vi "Teleop.vi"(10 "Match Info":T1={"Autonomous Elapsed Seconds"=0.0, "TeleOp Elapsed Seconds"=0.0, "Disabled Elapsed Seconds"=0.0, "Visited Autonomous"=FALSE, "Visited TeleOp"=FALSE, "Visited Disabled"=FALSE, "Autonomous Settings"={"Autonomous Style"=enum."Independent", "VI Refnum"=refnum}}, 11 "Call Context":T2) -> ()   [LabVIEW 2011]
doc: "This VI is called for each TeleOp packet received from the DS where the robot is not disabled. It is often used to read from the joysticks and update I/O or to update setpoints for timed control loops. It should complete and return within 20 milliseconds or it may miss DS packets."
uses:
  <vilib>/Rock Robotics/WPI/DriverStation/WPI_DriverStationDerivedRobotMode.ctl
  <vilib>/Rock Robotics/WPI/DriverStation/WPI_DriverStationMatch Info.ctl
  Robot Global Data.vi
panel:
  out "Position 4":dbl
  out "Position 3":dbl
  out "Shift Control":dbl=2.0 format="%.2f"
  in  "Left High":dbl=0.2
  in  "Right High":dbl=0.8
  in  "Left Mid":dbl=0.25
  in  "Right Mid":dbl=0.7
  in  "Shift Input 2":dbl
  in  "Left Low":dbl=0.8
  in  "Right Low":dbl=0.4
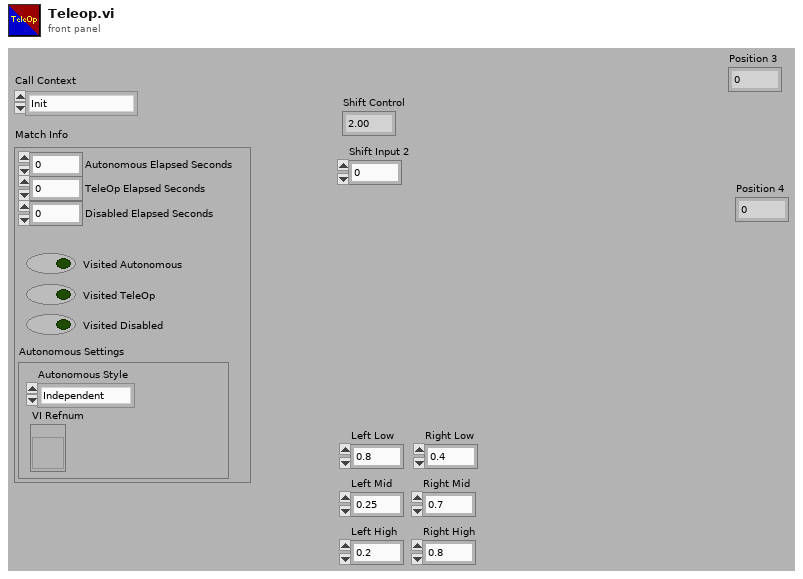
[diagram p1: front panel]
types:
  T1 = typedef "WPI_DriverStationMatch Info.ctl" = cluster{"Autonomous Elapsed Seconds":dbl, "TeleOp Elapsed Seconds":dbl, "Disabled Elapsed Seconds":dbl, "Visited Autonomous":bool, "Visited TeleOp":bool, "Visited Disabled":bool, "Autonomous Settings":cluster{"Autonomous Style":enum16{"Iterative", "Independent"}, "VI Refnum":refnum<vi>}}
  T2 = typedef "WPI_DriverStationDerivedRobotMode.ctl" = enum16{"Init", "Execute", "Stop"}
  T3 = typedef "WPI_MotorControlDeviceRef.ctl" = cluster{"DeviceStatus":errorcluster, "Type":enum16{"PWM", "CAN"}, "PWM":cluster{"Digital Module":T4, "PWM Channel":T5, "DeadBand":T6}, "CAN":cluster{"Device Number":u8, "Control Mode":T7, "Semaphore":T8, "Max Vout":dbl}, "Invert":bool, "TransformRef":T9, "InvTransformRef":T9}
  T4 = typedef "FPGA_TypedefDigitalModule.ctl" = enum16{"Digital Module 1", "Digital Module 2"}
  T5 = typedef "FPGA_DIOPWMChannel.ctl" = enum8{"PWM 1", "PWM 2", "PWM 3", "PWM 4", "PWM 5", "PWM 6", "PWM 7", "PWM 8", "PWM 9", "PWM 10", "Invalid"}
  T6 = typedef "WPI_PWMDeadband.ctl" = cluster{"Name":string, "maxPositivePwm":i32, "minPositivePwm":i32, "centerPwm":i32, "maxNegativePwm":i32, "minNegativePwm":i32, "angularRange":u16}
  T7 = typedef "WPI_CANJaguar_ControlMode.ctl" = enum8{"Percent VBus", "Current", "Speed", "Position", "Voltage"}
  T8 = typedef "Semaphore RefNum" = refnum<k1>
  T9 = typedef "WPI_PWMTransform_ConPane.ctl" = refnum<vi>
  T10 = typedef "WPI_JoystickDevRef.ctl" = cluster{"Device":T11}
  T11 = typedef "WPI_JoystickDeviceEnum.ctl" = enum16{"USB 1", "USB 2", "USB 3", "USB 4", "Kinect 1", "Kinect 2"}
  T12 = typedef "WPI_JoystickButtonState.ctl" = cluster{"Button 1":bool, "Button 2":bool, "Button 3":bool, "Button 4":bool, "Button 5":bool, "Button 6":bool, "Button 7":bool, "Button 8":bool, "Button 9":bool, "Button 10":bool, "Button 11":bool, "Button 12":bool}
  T13 = cluster{"axis 1 (x)":dbl, "axis 2 (y)":dbl, "axis 3 (throttle)":dbl, "axis 4":dbl, "axis 5":dbl, "axis 6":dbl}
  T14 = typedef "WPI_DigitalInputDevRef.ctl" = cluster{"DevStatus":errorcluster, "DIO Channel":T15, "Digital Module":T4}
  T15 = typedef "FPGA_DIOChannel.ctl" = enum8{"DIO 1", "DIO 2", "DIO 3", "DIO 4", "DIO 5", "DIO 6", "DIO 7", "DIO 8", "DIO 9", "DIO 10", "DIO 11", "DIO 12", "DIO 13", "DIO 14", "Invalid"}
  T16 = typedef "WPI_ServoDeviceRef.ctl" = cluster{"DeviceStatus":errorcluster, "Digital Module":T4, "PWM Channel":T5, "DeadBand":T6}
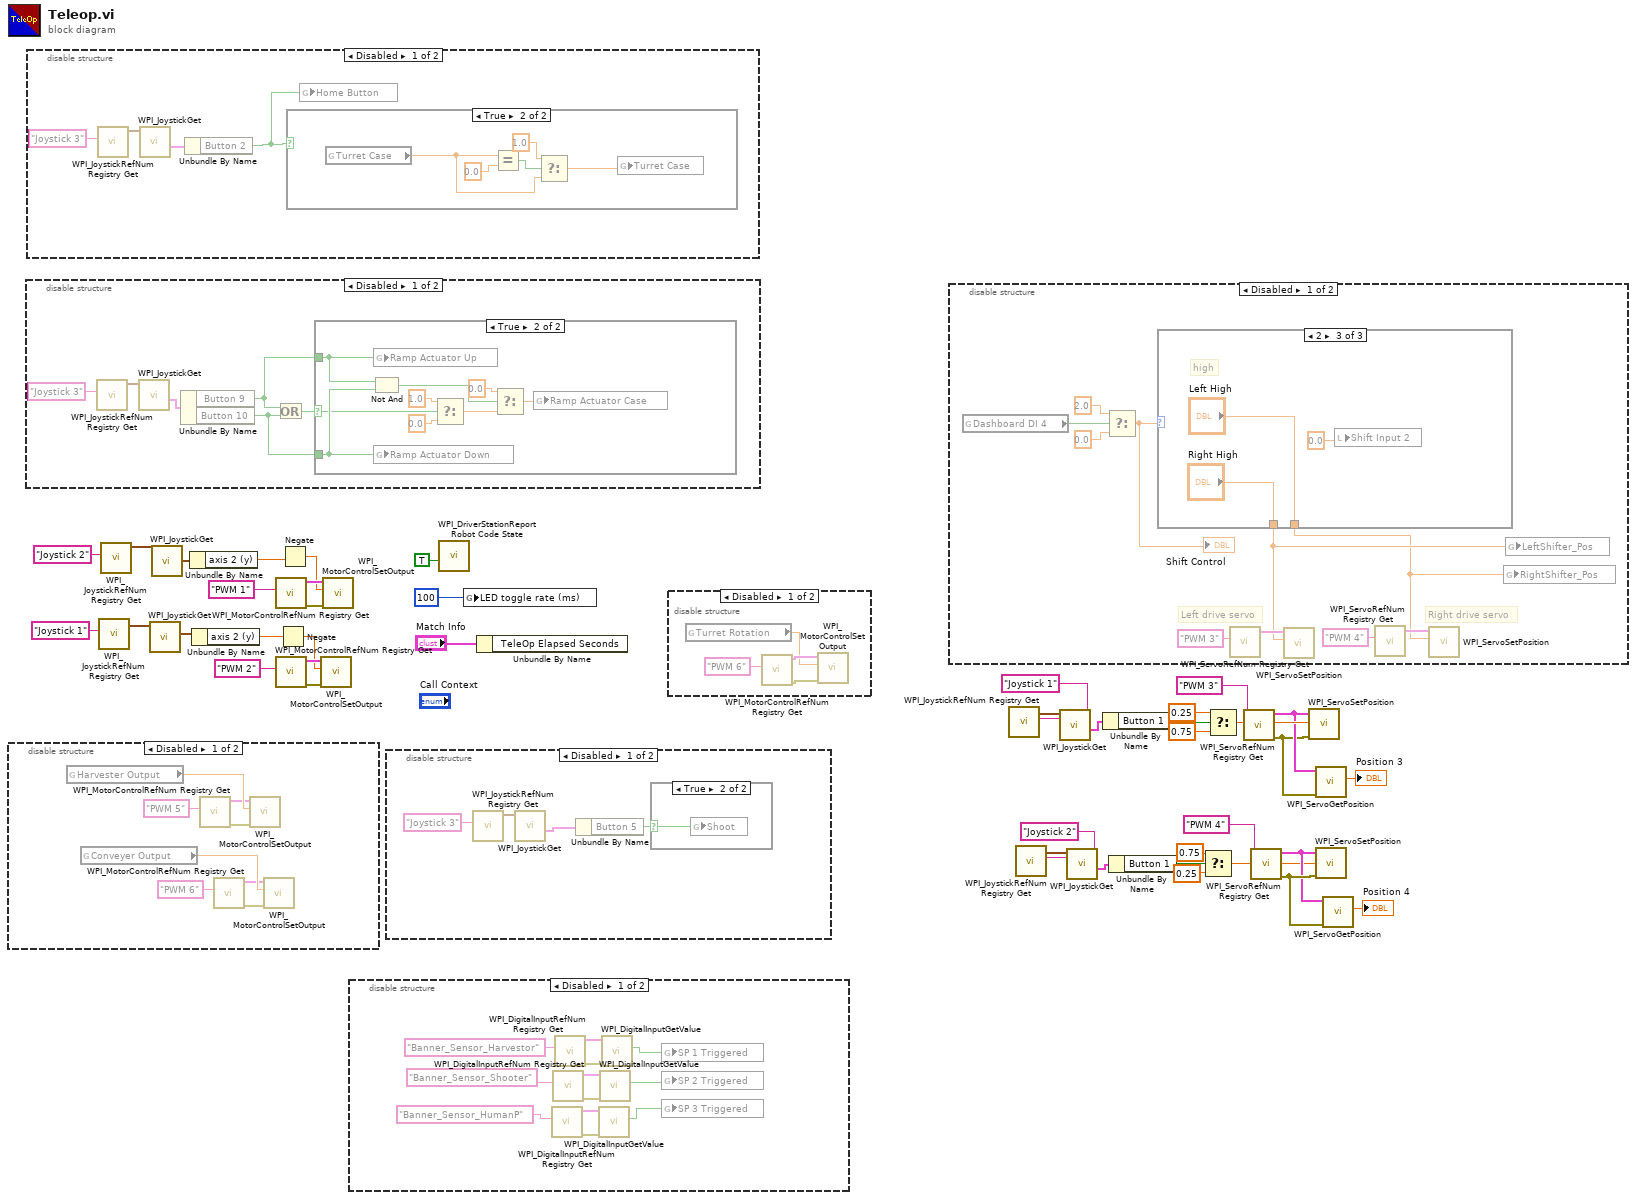
[diagram p0: block diagram]
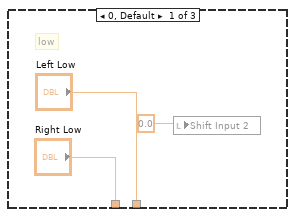
[diagram p11: hidden frame]
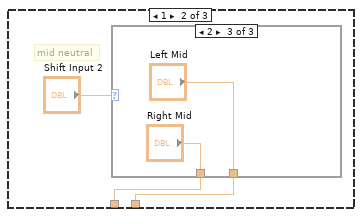
[diagram p12: hidden frame]
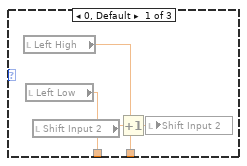
[diagram p13: hidden frame]
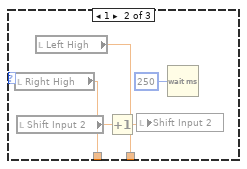
[diagram p14: hidden frame]
diagram:
  n1 = disable-structure shown="Disabled" {
    frame Disabled {
      n2 = global read "Robot Global Data.vi" "Harvester Output"() -> (w47:dbl)
      n3 = global read "Robot Global Data.vi" "Conveyer Output"() -> (w43:dbl)
      n4 = call <vilib>:"WPI_MotorControlRefNum Registry Get.vi"("refnum name"="PWM 5") -> ("error out"=w48:errorcluster, "MotorControlDevRef"=w46:T3)  [unwired: 9 in]
      n5 = call <vilib>:"WPI_MotorControlRefNum Registry Get.vi"("refnum name"="PWM 6") -> ("error out"=w44:errorcluster, "MotorControlDevRef"=w42:T3)  [unwired: 9 in]
      n6 = call <vilib>:"WPI_MotorControlSetOutput.vi"("error in (no error)"=w48, "Output"=w47, "MotorControlDevRef"=w46) -> ()  [unwired: 7 in, 2 out]
      n7 = call <vilib>:"WPI_MotorControlSetOutput.vi"("error in (no error)"=w44, "Output"=w43, "MotorControlDevRef"=w42) -> ()  [unwired: 7 in, 2 out]
    }
    frame Enabled {
    }
  }
  n8 = disable-structure shown="Disabled" {
    frame Disabled {
      n9 = call <vilib>:"WPI_JoystickRefNum Registry Get.vi"("refnum name"="Joystick 3") -> ("JoystickDevRef"=w55:T10)  [unwired: 9 in, 1 out]
      n10 = call <vilib>:"WPI_JoystickGet.vi"("JoystickDevRef"=w55) -> ("Buttons"=w54:T12)  [unwired: 4 in, 2 out]
      n11 = Unbundle By Name(w54) -> ("Button 9"=w52:bool, "Button 10"=w51:bool)
      n12 = Or(x=w52, y=w51) -> (x .or. y?=w50:bool)
      n13 = case shown="True" w50 {
        selector: w50 -> [_ w56]
        tunnel: w52 -> [_ w58]
        tunnel: w51 -> [_ w57]
        frame False {
        }
        frame True {
          n14 = Not And(1:w57, 2:w58) -> (0:w59:bool)
          n15 = global write "Robot Global Data.vi" "Ramp Actuator Up"(w58) -> ()
          n16 = global write "Robot Global Data.vi" "Ramp Actuator Down"(w57) -> ()
          n17 = Select(t=1.0, s=w56, f=0.0) -> (s? t:f=w61:dbl)
          n18 = Select(t=0.0, s=w59, f=w61) -> (s? t:f=w64:dbl)
          n19 = global write "Robot Global Data.vi" "Ramp Actuator Case"(w64) -> ()
        }
      }
    }
    frame Enabled {
    }
  }
  n20 = disable-structure shown="Disabled" {
    frame Disabled {
      n21 = call <vilib>:"WPI_JoystickRefNum Registry Get.vi"("refnum name"="Joystick 3") -> ("JoystickDevRef"=w66:T10)  [unwired: 9 in, 1 out]
      n22 = call <vilib>:"WPI_JoystickGet.vi"("JoystickDevRef"=w66) -> ("Buttons"=w67:T12)  [unwired: 4 in, 2 out]
      n23 = Unbundle By Name(w67) -> ("Button 2"=w65:bool)
      n24 = case shown="True" w65 {
        frame False {
        }
        frame True {
          n25 = global read "Robot Global Data.vi" "Turret Case"() -> (w70:dbl)
          n26 = Equal?(x=w70, y=0.0) -> (x = y?=w72:bool)
          n27 = Select(t=1.0, s=w72, f=w70) -> (s? t:f=w69:dbl)
          n28 = global write "Robot Global Data.vi" "Turret Case"(w69) -> ()
        }
      }
      n29 = global write "Robot Global Data.vi" "Home Button"(w65) -> ()
    }
    frame Enabled {
    }
  }
  n30 = call <vilib>:"WPI_JoystickRefNum Registry Get.vi"("refnum name"="Joystick 1") -> ("JoystickDevRef"=w33:T10)  [unwired: 9 in, 1 out]
  n31 = call <vilib>:"WPI_JoystickRefNum Registry Get.vi"("refnum name"="Joystick 2") -> ("JoystickDevRef"=w36:T10)  [unwired: 9 in, 1 out]
  n32 = call <vilib>:"WPI_JoystickGet.vi"("JoystickDevRef"=w33) -> ("Axes"=w37:T13)  [unwired: 4 in, 2 out]
  n33 = call <vilib>:"WPI_JoystickGet.vi"("JoystickDevRef"=w36) -> ("Axes"=w38:T13)  [unwired: 4 in, 2 out]
  n34 = Unbundle By Name(w38) -> ("axis 2 (y)"=w26:dbl)
  n35 = Unbundle By Name(w37) -> ("axis 2 (y)"=w24:dbl)
  n36 = call <vilib>:"WPI_MotorControlRefNum Registry Get.vi"("refnum name"="PWM 1") -> ("error out"=w30:errorcluster, "MotorControlDevRef"=w29:T3)  [unwired: 9 in]
  n37 = call <vilib>:"WPI_MotorControlRefNum Registry Get.vi"("refnum name"="PWM 2") -> ("error out"=w32:errorcluster, "MotorControlDevRef"=w31:T3)  [unwired: 9 in]
  n38 = Negate(x=w24) -> (-x=w23:dbl)
  n39 = Negate(x=w26) -> (-x=w25:dbl)
  n40 = call <vilib>:"WPI_MotorControlSetOutput.vi"("error in (no error)"=w32, "Output"=w23, "MotorControlDevRef"=w31) -> ()  [unwired: 7 in, 2 out]
  n41 = call <vilib>:"WPI_MotorControlSetOutput.vi"("error in (no error)"=w30, "Output"=w25, "MotorControlDevRef"=w29) -> ()  [unwired: 7 in, 2 out]
  n42 = disable-structure shown="Disabled" {
    frame Disabled {
      n43 = call <vilib>:"WPI_DigitalInputRefNum Registry Get.vi"("refnum name"="Banner_Sensor_HumanP") -> ("error out"=w80:errorcluster, "DigitalInputDevRef"=w79:T14)  [unwired: 9 in]
      n44 = call <vilib>:"WPI_DigitalInputRefNum Registry Get.vi"("refnum name"="Banner_Sensor_Shooter") -> ("error out"=w81:errorcluster, "DigitalInputDevRef"=w82:T14)  [unwired: 9 in]
      n45 = call <vilib>:"WPI_DigitalInputRefNum Registry Get.vi"("refnum name"="Banner_Sensor_Harvestor") -> ("error out"=w85:errorcluster, "DigitalInputDevRef"=w84:T14)  [unwired: 9 in]
      n46 = call <vilib>:"WPI_DigitalInputGetValue.vi"("error in (no error)"=w80, "DigitalInputDevRef"=w79) -> ("Value"=w77:bool)  [unwired: 7 in, 2 out]
      n47 = call <vilib>:"WPI_DigitalInputGetValue.vi"("error in (no error)"=w81, "DigitalInputDevRef"=w82) -> ("Value"=w78:bool)  [unwired: 7 in, 2 out]
      n48 = call <vilib>:"WPI_DigitalInputGetValue.vi"("error in (no error)"=w85, "DigitalInputDevRef"=w84) -> ("Value"=w83:bool)  [unwired: 7 in, 2 out]
      n49 = global write "Robot Global Data.vi" "SP 1 Triggered"(w83) -> ()
      n50 = global write "Robot Global Data.vi" "SP 2 Triggered"(w78) -> ()
      n51 = global write "Robot Global Data.vi" "SP 3 Triggered"(w77) -> ()
    }
    frame Enabled {
    }
  }
  n52 = disable-structure shown="Disabled" {
    frame Disabled {
      n53 = call <vilib>:"WPI_JoystickRefNum Registry Get.vi"("refnum name"="Joystick 3") -> ("JoystickDevRef"=w87:T10)  [unwired: 9 in, 1 out]
      n54 = call <vilib>:"WPI_JoystickGet.vi"("JoystickDevRef"=w87) -> ("Buttons"=w88:T12)  [unwired: 4 in, 2 out]
      n55 = Unbundle By Name(w88) -> ("Button 5"=w86:bool)
      n56 = case shown="True" w86 {
        selector: w86 -> [_ w90]
        frame False {
        }
        frame True {
          n57 = global write "Robot Global Data.vi" "Shoot"(w90) -> ()
        }
      }
    }
    frame Enabled {
    }
  }
  n58 = call <vilib>:"WPI_DriverStationReport Robot Code State.vi"("TeleOp"=TRUE ("Autonomous")) -> ()  [unwired: 10 in, 1 out]
  n59 = global write "Robot Global Data.vi" "LED toggle rate (ms)"(u32 100 ("LED ms toggle rate")) -> ()
  n60 = Unbundle By Name("Match Info") -> ()  [unwired: 1 out]
  n61 = disable-structure shown="Disabled" {
    frame Disabled {
      n62 = global read "Robot Global Data.vi" "Turret Rotation"() -> (w91:dbl)
      n63 = call <vilib>:"WPI_MotorControlRefNum Registry Get.vi"("refnum name"="PWM 6") -> ("error out"=w94:errorcluster, "MotorControlDevRef"=w93:T3)  [unwired: 9 in]
      n64 = call <vilib>:"WPI_MotorControlSetOutput.vi"("error in (no error)"=w94, "Output"=w91, "MotorControlDevRef"=w93) -> ()  [unwired: 7 in, 2 out]
    }
    frame Enabled {
    }
  }
  n65 = disable-structure shown="Disabled" {
    frame Disabled {
      # "Right drive servo"
      # "Left drive servo"
      n66 = global read "Robot Global Data.vi" "Dashboard DI 4"() -> (w97:bool)
      n67 = Select(t=2.0, s=w97, f=0.0) -> (s? t:f=w99:dbl)
      "Shift Control" <- w99
      n68 = case shown="2" w99 {
        tunnel: ["Left Low" w109 "Left High"] -> w95
        tunnel: ["Right Low" w108 "Right High"] -> w96
        frame 0, Default {
          # "low"
          n69 = local write "Shift Input 2"(0.0 ("Input 2")) -> ()
        }
        frame 1 {
          # "mid neutral"
          n70 = case shown="2" "Shift Input 2" {
            tunnel: [w114 w115 "Left Mid"] -> w109
            tunnel: [w113 w116 "Right Mid"] -> w108
            frame 0, Default {
              n71 = local read "Left High"() -> (w114:dbl)
              n72 = local read "Left Low"() -> (w113:dbl)
              n73 = local read "Shift Input 2"() -> (w112:dbl)
              n74 = Increment(x=w112) -> (x+1=w111:dbl)
              n75 = local write "Shift Input 2"(w111) -> ()
            }
            frame 1 {
              n76 = local read "Right High"() -> (w116:dbl)
              n77 = local read "Shift Input 2"() -> (w118:dbl)
              n78 = local read "Left High"() -> (w115:dbl)
              n79 = Increment(x=w118) -> (x+1=w117:dbl)
              n80 = local write "Shift Input 2"(w117) -> ()
              n81 = Wait (ms)(milliseconds to wait=u32 250) -> ()  [unwired: 1 out]
            }
            frame 2 {
            }
          }
        }
        frame 2 {
          # "high"
          n82 = local write "Shift Input 2"(0.0 ("Input 2")) -> ()
        }
      }
      n83 = call <vilib>:"WPI_ServoRefNum Registry Get.vi"("refnum name"="PWM 3") -> ("ServoDeviceRef"=w104:T16)  [unwired: 1 in, 9 out]
      n84 = call <vilib>:"WPI_ServoSetPosition.vi"("Position"=w96, "ServoDeviceRef"=w104) -> ()  [unwired: 1 in, 9 out]
      n85 = call <vilib>:"WPI_ServoRefNum Registry Get.vi"("refnum name"="PWM 4") -> ("ServoDeviceRef"=w100:T16)  [unwired: 1 in, 9 out]
      n86 = call <vilib>:"WPI_ServoSetPosition.vi"("Position"=w95, "ServoDeviceRef"=w100) -> ()  [unwired: 1 in, 9 out]
      n87 = global write "Robot Global Data.vi" "RightShifter_Pos"(w95) -> ()
      n88 = global write "Robot Global Data.vi" "LeftShifter_Pos"(w96) -> ()
    }
    frame Enabled {
    }
  }
  n89 = call <vilib>:"WPI_JoystickRefNum Registry Get.vi"("refnum name"="Joystick 1") -> ("JoystickDevRef"=w22:T10)  [unwired: 9 in, 1 out]
  n90 = call <vilib>:"WPI_JoystickRefNum Registry Get.vi"("refnum name"="Joystick 2") -> ("JoystickDevRef"=w1:T10)  [unwired: 9 in, 1 out]
  n91 = call <vilib>:"WPI_JoystickGet.vi"("JoystickDevRef"=w22) -> ("Buttons"=w20:T12)  [unwired: 4 in, 2 out]
  n92 = call <vilib>:"WPI_JoystickGet.vi"("JoystickDevRef"=w1) -> ("Buttons"=w3:T12)  [unwired: 4 in, 2 out]
  n93 = Unbundle By Name(w20) -> ("Button 1"=w19:bool)
  n94 = Unbundle By Name(w3) -> ("Button 1"=w4:bool)
  n95 = Select(t=0.75, s=w4, f=0.25) -> (s? t:f=w7:dbl)
  n96 = Select(t=0.25, s=w19, f=0.75) -> (s? t:f=w16:dbl)
  n97 = call <vilib>:"WPI_ServoRefNum Registry Get.vi"("refnum name"="PWM 3") -> ("error out"=w13:errorcluster, "ServoDeviceRef"=w14:T16)  [unwired: 9 in]
  n98 = call <vilib>:"WPI_ServoRefNum Registry Get.vi"("refnum name"="PWM 4") -> ("error out"=w10:errorcluster, "ServoDeviceRef"=w9:T16)  [unwired: 9 in]
  n99 = call <vilib>:"WPI_ServoSetPosition.vi"("error in (no error)"=w13, "Position"=w16, "ServoDeviceRef"=w14) -> ()  [unwired: 7 in, 2 out]
  n100 = call <vilib>:"WPI_ServoGetPosition.vi"("error in (no error)"=w13, "ServoDeviceRef"=w14) -> ("Position"=→"Position 3":dbl)  [unwired: 7 in, 2 out]
  n101 = call <vilib>:"WPI_ServoSetPosition.vi"("error in (no error)"=w10, "Position"=w7, "ServoDeviceRef"=w9) -> ()  [unwired: 7 in, 2 out]
  n102 = call <vilib>:"WPI_ServoGetPosition.vi"("error in (no error)"=w10, "ServoDeviceRef"=w9) -> ("Position"=→"Position 4":dbl)  [unwired: 7 in, 2 out]
